vi "UI_solvePuzzle.vi"(8 "error in (no error)":errorcluster) -> (0 "error out":errorcluster, 3 "String OUT":string)   [LabVIEW 2020]
panel:
  in  "Accept":bool
  in  "String":string
  # "Solve the Puzzle:"
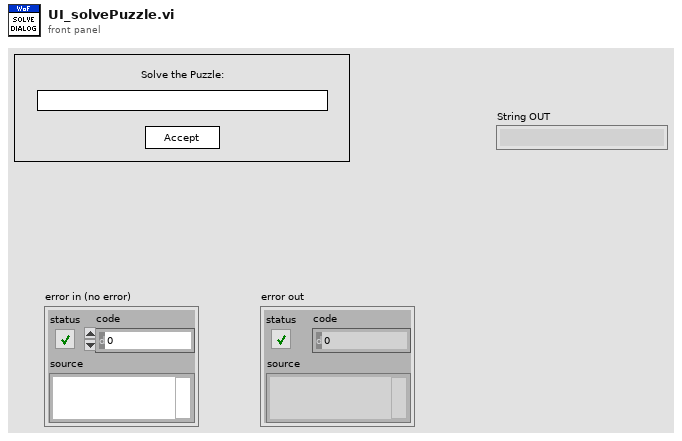
[diagram p1: front panel]
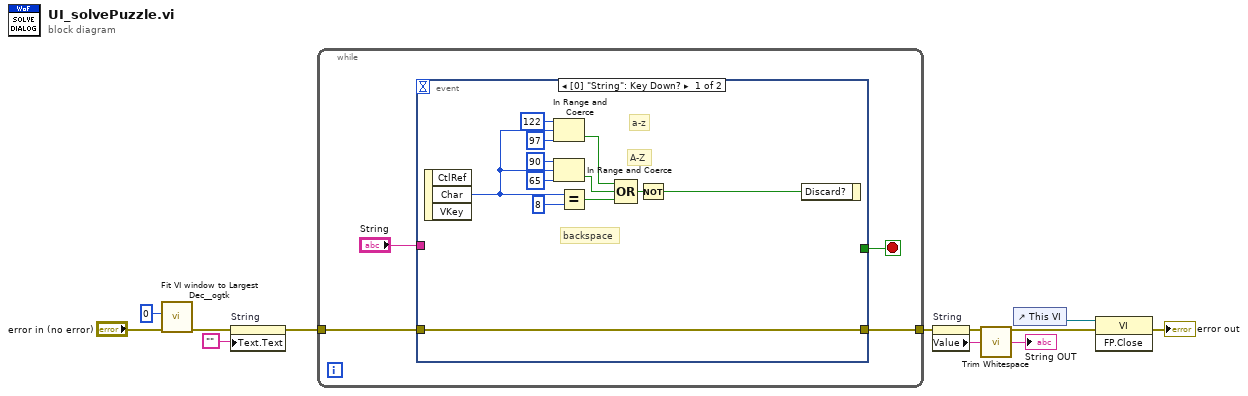
[diagram p0: block diagram]
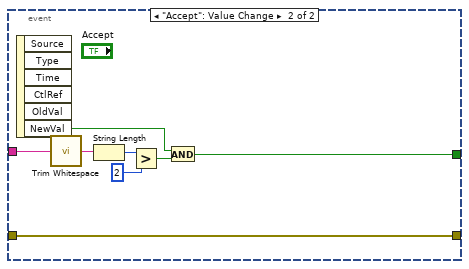
[diagram p2: hidden frame]
diagram:
  n1 = call <userlib>:"Fit VI window to Largest Dec__ogtk.vi"("error in (no error)"="error in (no error)", "border spacing (2 px)"=0) -> ("error out"=w9:errorcluster)  [unwired: 4 in, 1 out]
  n2 = property on="String" class="Str"(error in=w9, "Text.Text"="") -> (error out=w11:errorcluster)  [unwired: 1 in, 1 out]
  n3 = while {
    tunnel: w11 -> [w13]
    tunnel: [w12] -> w7
    stop <- w15 stop-if-true
    n4 = event shown="[0] \"String\": Key Down?" {
      selector: _ -> [_ _]
      dyn-events: _ -> [_ _]
      timeout: _ -> [_ _]
      tunnel: [_ w29] -> w15
      tunnel: "String" -> [_ w34]
      tunnel: w13 -> [w16 w28]
      tunnel: [w16 w28] -> w12
      event "String": Key Down? {
        # "backspace"
        # "A-Z"
        # "a-z"
        n5 = event-data() -> ("Char"=w23:i16)  [unwired: 1 in, 2 out]
        n6 = In Range and Coerce(upper limit=i16 122, x=w23, lower limit=i16 97) -> (In Range?=w19:bool)  [unwired: 1 out]
        n7 = In Range and Coerce(upper limit=i16 90, x=w23, lower limit=i16 65) -> (In Range?=w20:bool)  [unwired: 1 out]
        n8 = Equal?(x=w23, y=i16 8) -> (x = y?=w21:bool)
        n9 = Compound Arithmetic op=OR(w19, w20, w21) -> (w18:bool)
        n10 = Not(x=w18) -> (.not. x?=w17:bool)
        n11 = event-data("Discard?"=w17) -> ()  [unwired: 1 in, 1 out]
      }
      event "Accept": Value Change {
        n12 = event-data() -> ("NewVal"=w31:bool)  [unwired: 1 in, 5 out]
        n13 = call <vilib>:"Trim Whitespace.vi"("string"=w34) -> ("trimmed string"=w35:string)  [unwired: 1 in]
        n14 = String Length(string=w35) -> (length=w33:i32)
        n15 = Greater?(x=w33, y=2) -> (0:w30:bool)
        n16 = And(x=w31, y=w30) -> (x .and. y?=w29:bool)
      }
    }
  }
  n17 = property on="String" class="Str"(error in=w7) -> (error out=w3:errorcluster, "Value"=w6:string)  [unwired: 1 in, 1 out]
  n18 = call <vilib>:"Trim Whitespace.vi"("string"=w6) -> ("trimmed string"=→"String OUT":string)  [unwired: 1 in]
  n19 = control-ref of="This VI"() -> (w2:refnum<vi>)
  n20 = invoke class="VI" method="FP.Close"(reference=w2, error in=w3) -> (error out=→"error out":errorcluster)  [unwired: 1 in, 2 out]
